vi "Send Start Recipe.vi"(7 "Message Priority (Normal)":T1=enum."Normal", 8 "error in (no error)":errorcluster, 10 "Recipe File":path, 11 "Interlock Q Class":refnum<class "Interlock Q Class.lvclass">) -> (0 "error out":errorcluster, 3 "Interlock Q Class":refnum<class "Interlock Q Class.lvclass">)   [LabVIEW 2022 SP3, in "Recipe Process.lvlib" / "Start Recipe Msg.lvclass"]
doc: "This VI sends the message to an actor."
uses:
  Start Recipe Msg.lvclass
  <vilib>/ActorFramework/Message Enqueuer/Message Priority.ctl
  Start Recipe Msg.lvclass/Start Recipe Msg.ctl
  <vilib>/ActorFramework/Message Enqueuer/Message Enqueuer.lvclass/Message Enqueuer.ctl
  <vilib>/ActorFramework/Message Priority Queue/Priority Enqueue.vi
  XY Stage/Process Actor/Process Framework/Interlock Q Class/Interlock Q Class.lvclass
  C:/Program Files/National Instruments/LabVIEW 2022/vi.lib/ActorFramework/Message/Message.lvclass
  C:/XY Stage/Process Actor Project/Recipe Process/Recipe Process Messages/Start Recipe Msg/Start Recipe Msg.lvclass
  <vilib>/ActorFramework/Message Enqueuer/Message Enqueuer.lvclass
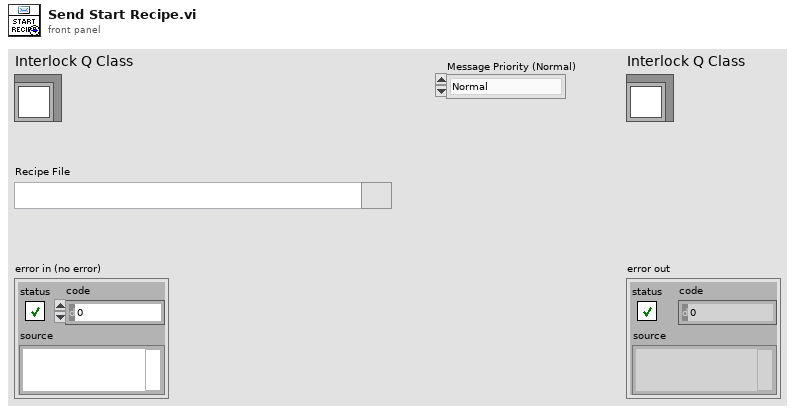
[diagram p1: front panel]
types:
  T1 = typedef "Actor Framework.lvlib/Message Enqueuer.lvclass/Message Priority.ctl" = enum16{"Low", "Normal", "High"}
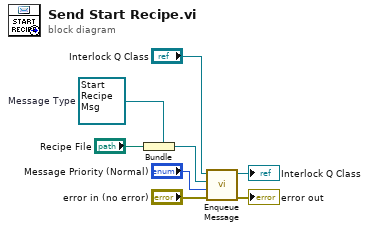
[diagram p0: block diagram]
diagram:
  w8 = refnum<class "Start Recipe Msg.lvclass"> refnum  # Message Type
  n1 = Bundle(cluster=w8, "Recipe File") -> (w4:refnum<class "Start Recipe Msg.lvclass">)
  n2 = call-dynamic "Enqueue Message.vi"("error in (no error)"="error in (no error)", "Message Priority (Normal)"="Message Priority (Normal)", "Message"=w4, "Interlock Q Class in"="Interlock Q Class") -> ("error out"=→"error out":errorcluster, "Interlock Q Class out"=→"Interlock Q Class":refnum<class "Interlock Q Class.lvclass">)  [unwired: 6 in]
